vi "格式化时间.vi"() -> ()   [LabVIEW 2022 SP3]
doc: "本VI是为《我和LabVIEW》一书编写的示例。\n关于本书的介绍请参考网页：\nhttp://ruanqizhen.spaces.live.com/blog/cns!5852D4F797C53FB6!4310.entry"
panel:
  out "时间标识":timestamp
  out "时间字符串":string
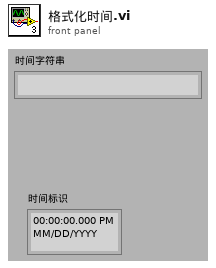
[diagram p1: front panel]
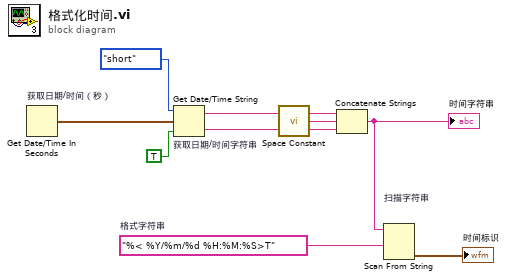
[diagram p0: block diagram]
diagram:
  w1 = "%< %Y/%m/%d %H:%M:%S>T"  # 格式字符串
  n1 = Get Date/Time In Seconds "获取日期/时间（秒）"() -> (seconds since 1Jan1904=w8:timestamp)
  n2 = Get Date/Time String "获取日期/时间字符串"(date format (0)=enum16{"short", "long", "abbreviated"}."short" ("日期格式(0)"), seconds (now)=w8, want seconds? (F)=TRUE ("需要秒？(F)")) -> (date string=w7:string, time string=w5:string)
  n3 = call <vilib>:"Space Constant.vi"() -> ("String"=w4:string)
  n4 = Concatenate Strings(w7, w4, w5) -> (w3:string)
  "时间字符串" <- w3
  n5 = Scan From String "扫描字符串"(format string=w1, input string=w3) -> (output 1=→"时间标识":timestamp)  [unwired: 2 in, 4 out]
